vi "ROI grp-Case-Delete selected POI.vi"(8 "error in (no error)":errorcluster) -> (0 "error out":errorcluster)   [LabVIEW 2013]
uses:
  Globals/gl_ROI grp window globals.vi
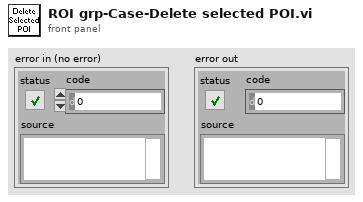
[diagram p1: front panel]
types:
  T1 = cluster{"Caption-Right button":string, "Caption-Left button":string, "Message to display":string, "Delay before close":u32, "Window Colour":u32, "Cancel button disabled?":enum8{"Enabled", "Disabled", "Disabled and Grayed Out"}}
  T2 = enum8{"Enabled", "Disabled", "Disabled and Grayed Out"}
  T3 = typedef "ROI grp-window ctrl refs.ctl" = cluster{"This VI":refnum<vi>, "Pane":refnum<vi>, "Table":refnum<vi>}
  T4 = cluster{"Group index":i32, "ROI numbers deleted":i32[]}[]
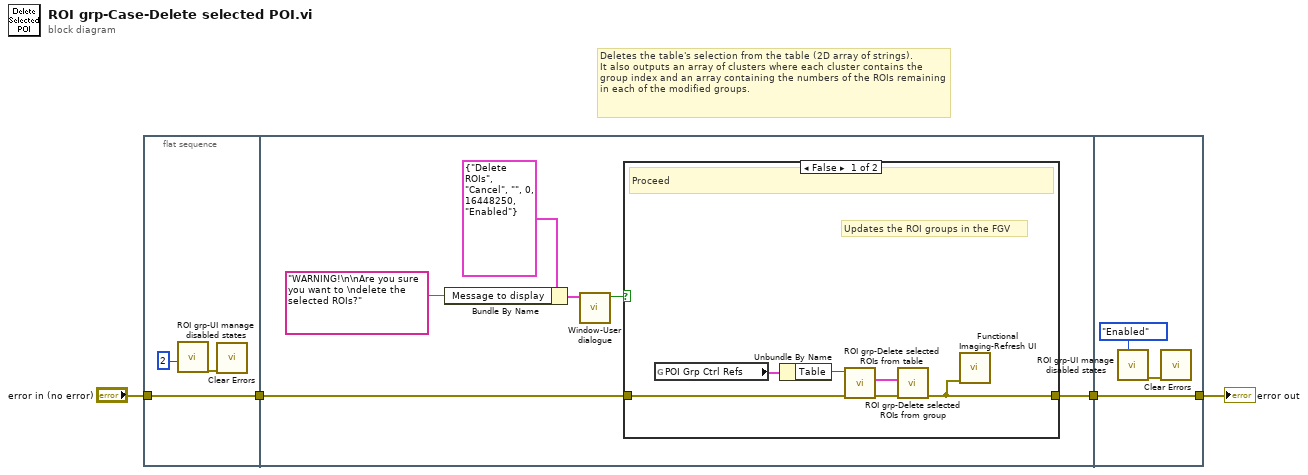
[diagram p0: block diagram]
diagram:
  # "Deletes the table's selection from the table (2D array of strings).\nIt also outputs an array of clusters where each cluster contains the group index and an array containing the numbers of the ROIs remaining in each of the modified groups."
  n1 = flat-sequence {
    tunnel: "error in (no error)" -> [w5]
    tunnel: [w5] -> w1
    tunnel: [w9] -> w3
    tunnel: w1 -> [w8]
    tunnel: [w20] -> w4
    tunnel: w3 -> [w20]
    frame #0 {
      n2 = call "ROI grp-UI manage disabled states.vi"("UI elemente enabled?"=2) -> ("error out"=w6:errorcluster)  [unwired: 10 in]
      n3 = call <vilib>:"Clear Errors.vi"("error in (no error)"=w6) -> ()  [unwired: 6 in, 1 out]
    }
    frame #1 {
      n4 = Bundle By Name(cluster=T1 {"Caption-Right button"="Delete ROIs", "Caption-Left button"="Cancel", "Message to display"="", "Delay before close"=0, "Window Colour"=16448250, "Cancel button disabled?"=enum."Enabled"} ("Input cluster"), "Message to display"="WARNING!\n\nAre you sure you want to \ndelete the selected ROIs?" ("Message")) -> (w11:T1)
      n5 = call "Window-User dialogue.vi"("Input cluster"=w11) -> ("Left Button (Cancel)"=w13:bool)  [unwired: 10 in]
      n6 = case shown="False" w13 {
        tunnel: w8 -> [w18 _]
        tunnel: [w15 _] -> w9
        frame False {
          # "Updates the ROI groups in the FGV"
          # "Proceed"
          n7 = global read "gl_ROI grp window globals.vi" "POI Grp Ctrl Refs"() -> (w17:T3)
          n8 = Unbundle By Name(w17) -> ("Table"=w19:refnum<vi>)
          n9 = call "ROI grp-Delete selected ROIs from table.vi"("error in (no error)"=w18, "Table in"=w19) -> ("error out"=w16:errorcluster, "ROI number of ROIs deleted from each group."=w14:T4)  [unwired: 7 in, 1 out]
          n10 = call "ROI grp-Delete selected ROIs from group.vi"("error in (no error)"=w16, "ROI number of ROIs deleted from each group."=w14) -> ("error out"=w15:errorcluster)  [unwired: 9 in]
          n11 = call "Functional Imaging-Refresh UI.vi"("error in (no error)"=w15) -> ()  [unwired: 11 in]
        }
        frame True {
          # "Cancelled"
        }
      }
    }
    frame #2 {
      n12 = call "ROI grp-UI manage disabled states.vi"("UI elemente enabled?"=T2."Enabled") -> ("error out"=w22:errorcluster)  [unwired: 10 in]
      n13 = call <vilib>:"Clear Errors.vi"("error in (no error)"=w22) -> ()  [unwired: 6 in, 1 out]
    }
  }
  "error out" <- w4
